vi "Read lockin.vi"(8 "error in (no error)":errorcluster, 11 "lockin in":refnum<class "system.lvclass">) -> (0 "error out":errorcluster, 2 "lockin":T4, 3 "lockin out":refnum<class "system.lvclass">)   [LabVIEW 2016, in "system.lvclass"]
uses:
  system.lvclass
  Typedefs/lockin_config.ctl
  Typedefs/input_signals.ctl
  Typedefs/lockin_results.ctl
  system.lvclass/system.ctl
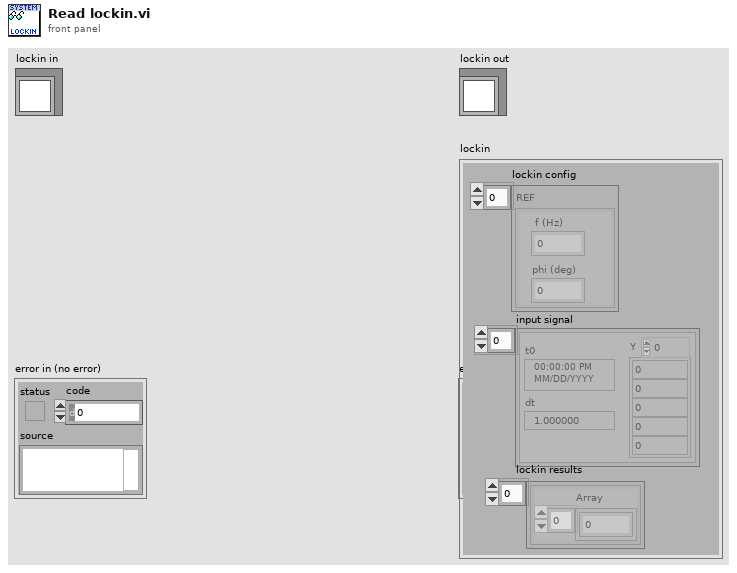
[diagram p1: front panel]
types:
  T1 = typedef "system.lvclass/lockin_config.ctl" = cluster{" f (Hz)":dbl, "phi (deg)":dbl}[]
  T2 = typedef "system.lvclass/input_signals.ctl" = waveform(dbl)[]
  T3 = typedef "system.lvclass/lockin_results.ctl" = cluster{"Array":dbl[]}[]
  T4 = cluster{"lockin config":T1, "input signal":T2, "lockin results":T3}
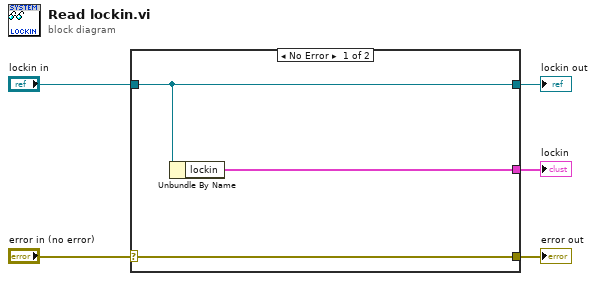
[diagram p0: block diagram]
diagram:
  n1 = case shown="No Error" "error in (no error)" {
    selector: "error in (no error)" -> [w8 w9]
    tunnel: [w8 w9] -> w4
    tunnel: [w7 w10] -> w2
    tunnel: "lockin in" -> [w7 w10]
    tunnel: [w6 _] -> w1
    frame No Error {
      n2 = Unbundle By Name(w7) -> ("lockin"=w6:T4)
    }
    frame Error {
    }
  }
  "error out" <- w4
  "lockin out" <- w2
  "lockin" <- w1
